vi "16 Bit Fletcher Checksum.vi"(8 "Error In":errorcluster, 11 "Input Array":u8[](array[numeric])) -> (0 "Error Out":errorcluster, 2 "B (LSB)":u8 format="%02x", 3 "A (MSB)":u8 format="%02x")   [LabVIEW 2012]
doc: "This VI calculates the MSB and LSB Fletcher Checksum."
panel:
  out "Number of Items in array":i32
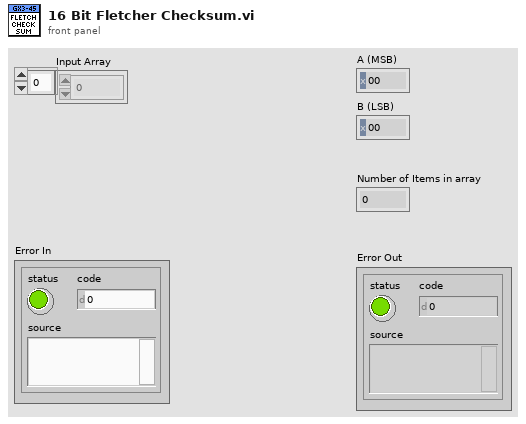
[diagram p1: front panel]
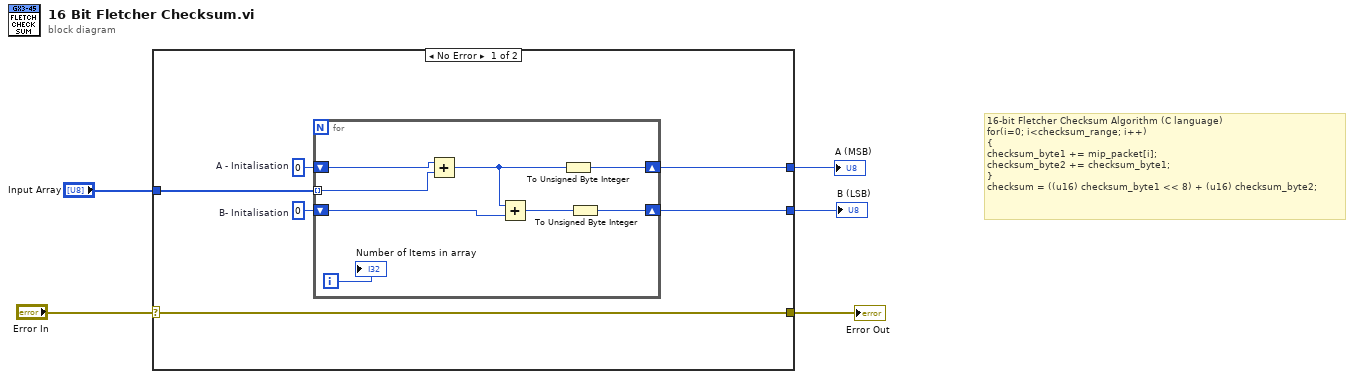
[diagram p0: block diagram]
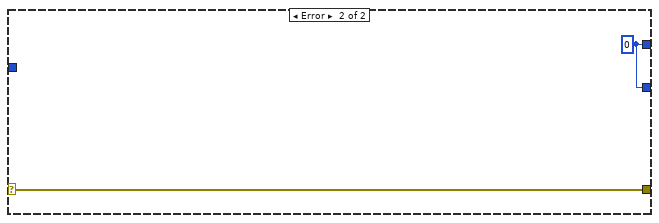
[diagram p2: hidden frame]
diagram:
  # "16-bit Fletcher Checksum Algorithm (C language)\nfor(i=0; i<checksum_range; i++)\n{\nchecksum_byte1 += mip_packet[i];\nchecksum_byte2 += checksum_byte1;\n}\nchecksum = ((u16) checksum_byte1 << 8) + (u16) checksum_byte2;"
  n1 = case shown="No Error" "Error In" {
    selector: "Error In" -> [w8 w21]
    tunnel: "Input Array" -> [w9 _]
    tunnel: [w8 w21] -> w3
    tunnel: [w7 w20] -> w2
    tunnel: [w6 w20] -> w1
    frame No Error {
      w10 = u8 0  # B- Initalisation
      w11 = u8 0  # A - Initalisation
      n2 = for {
        tunnel: w9 -> [w19] mode=indexing
        shift-right: [w16] -> w7
        shift-left: w11 -> [w18]
        shift-right: [w15] -> w6
        shift-left: w10 -> [w17]
        i -> [w14]
        n3 = Add(x=w18, y=w19) -> (x+y=w13:u8)
        n4 = Add(x=w13, y=w17) -> (x+y=w12:u8)
        n5 = To Unsigned Byte Integer(number=w13) -> (unsigned 8bit integer=w16:u8)
        n6 = To Unsigned Byte Integer(number=w12) -> (unsigned 8bit integer=w15:u8)
        "Number of Items in array" <- w14
      }
    }
    frame Error {
      w20 = u8 0 ("A - Initalisation")
    }
  }
  "Error Out" <- w3
  "A (MSB)" <- w2
  "B (LSB)" <- w1
